vi "Class to Variant.vi"(8 "error in (no error)":errorcluster, 10 "Data in":variant, 11 "VI Analyzer Node in":refnum<class "VI Analyzer Node.lvclass">) -> (0 "error out":errorcluster, 1 "Serialized Object Name":string, 2 "Data Out":variant, 3 "VI Analyzer Node out":refnum<class "VI Analyzer Node.lvclass">)   [LabVIEW 2014, in "VI Analyzer Node.lvclass"]
uses:
  VI Analyzer Node.lvclass
  Shared/Controls/VI Analyzer - STYP.ctl
  VI Analyzer Node.lvclass/VI Analyzer Node.ctl
  Classes/Build Job/Build Job.lvclass
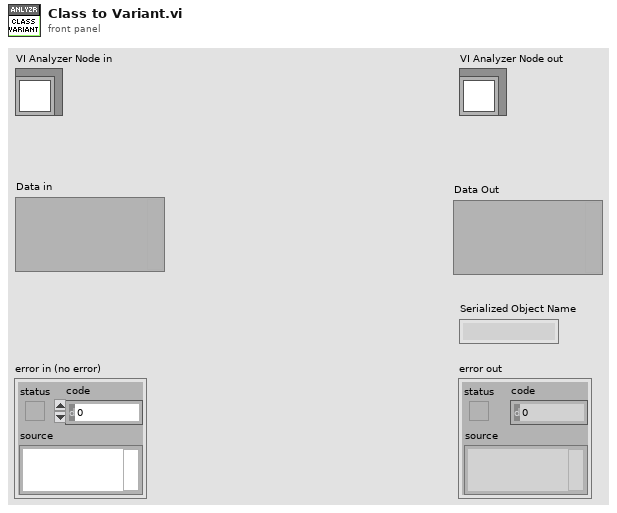
[diagram p1: front panel]
types:
  T1 = typedef "VI Analyzer - STYP.ctl" = cluster{"Executor_Number":string, "Workspace_Path":string, "Test File":string}
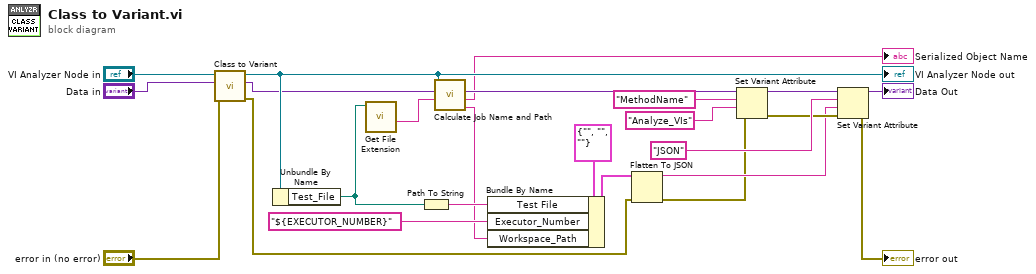
[diagram p0: block diagram]
diagram:
  n1 = call-parent "Class to Variant.vi"("error in (no error)"="error in (no error)", "Data in"="Data in", "Build Job in"="VI Analyzer Node in") -> ("error out"=w2:errorcluster, "Data Out"=w3:variant, "Build Job out"=w17:refnum<class "VI Analyzer Node.lvclass">)  [unwired: 5 in, 1 out]
  "VI Analyzer Node out" <- w17
  n2 = Unbundle By Name(w17) -> ("Test_File"=w18:path)
  n3 = call <vilib>:"Get File Extension.vi"("file"=w18) -> ("filename without extension"=w19:string)  [unwired: 7 in, 3 out]
  n4 = Path To String(path=w18) -> (string=w21:string)
  n5 = call "Calculate Job Name and Path.vi"("Job Target"=w19, "Data in"=w3, "Build Job"=w17) -> ("Workspace Path"=w1:string, "Job Name"=→"Serialized Object Name":string, "Data out"=w9:variant)  [unwired: 6 in]
  n6 = Bundle By Name(cluster=T1 {"Executor_Number"="", "Workspace_Path"="", "Test File"=""} ("VI Analyzer - STYP.ctl"), "Test File"=w21, "Executor_Number"="${EXECUTOR_NUMBER}", "Workspace_Path"=w1) -> (w6:T1)
  n7 = Flatten To JSON(anything=w6, error in (no error)=w2) -> (JSON string=w10:string, 11:w7:errorcluster)  [unwired: 1 in]
  n8 = Set Variant Attribute(Variant=w9, name="MethodName", value="Analyze_VIs", error in=w7) -> (Variant out=w13:variant, error out=w11:errorcluster)  [unwired: 1 out]
  n9 = Set Variant Attribute(Variant=w13, name="JSON" ("Name"), value=w10, error in=w11) -> (Variant out=→"Data Out":variant, error out=→"error out":errorcluster)  [unwired: 1 out]
